vi "ReadSweepConfigurationFile.vi"(8 "error in (no error)":errorcluster, 10 "Path":path, 11 "SweepControl in":refnum<class "SweepControl.lvclass">) -> (0 "error out":errorcluster, 2 "Data":variant, 3 "SweepControl out":refnum<class "SweepControl.lvclass">)   [LabVIEW 2016, in "SweepControl.lvclass"]
uses:
  SweepControl.lvclass
  Transport/subVI/LockinVsg Configuration--Cluster.ctl
  Typedefs/Continuous B Sweep Configuration--Cluster.ctl
  Typedefs/Enum - Experiments.ctl
  Typedefs/Sweep Control Configuration--Cluster.ctl
  Typedefs/ScanControl.ctl
  Typedefs/Cluster - ScanControl.ctl
  Typedefs/Enum - Priority.ctl
  Typedefs/Enum - Action.ctl
  Typedefs/ScanParamters.ctl
  Typedefs/Cluster - ScanParamters.ctl
  <vilib>/addons/_JKI.lib/Serialization/JSON/JKI JSON Serialization.lvlib
  Transport/Transport.lvclass
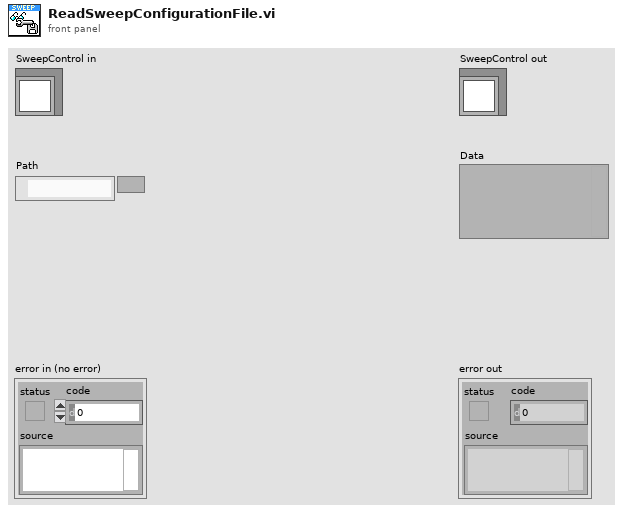
[diagram p1: front panel]
types:
  T1 = typedef "Transport.lvclass/LockinVsg Configuration--Cluster.ctl" = cluster{"Vsg Values":dbl[]}
  T2 = typedef "SweepControl.lvclass/Continuous B Sweep Configuration--Cluster.ctl" = cluster{"B field values":dbl[], "Experiment":T3}
  T3 = typedef "SweepControl.lvclass/Enum - Experiments.ctl" = enum16{"IV", "Lockin_time", "Lockin_Vsg", "Lockin (experimental)", "Lockin_Vsg_JKISM"}
  T4 = typedef "SweepControl.lvclass/Sweep Control Configuration--Cluster.ctl" = cluster{"Scan control":T5, "Scan parameters":T9, "Experiment":T3}
  T5 = typedef "SweepControl.lvclass/ScanControl.ctl" = T6[]
  T6 = typedef "SweepControl.lvclass/Cluster - ScanControl.ctl" = cluster{"Priority":T7, "Scan name":T8}
  T7 = typedef "SweepControl.lvclass/Enum - Priority.ctl" = enum16{"Priority 0", "Priority 1", "Priority 2", "Priority 3", "Priority 4", "Priority 5"}
  T8 = typedef "SweepControl.lvclass/Enum - Action.ctl" = enum16{"OFF", "DSA_Vamp", "DSA_freq", "DSA_Vsg1", "DSA_Vsg2", "DSA_Vsg3", "DAQ_Vbg", "B_Field", "Humidity", "Temp", "MW_freq1", "MW_freq2", "MW_amplitude1", "MW_amplitude2"}
  T9 = typedef "SweepControl.lvclass/ScanParamters.ctl" = T10[]
  T10 = typedef "SweepControl.lvclass/Cluster - ScanParamters.ctl" = cluster{"Start":dbl, "End":dbl, "Step":dbl, "Rate":dbl, "wait (ms)":u32, "Address":string, "channel":i32}
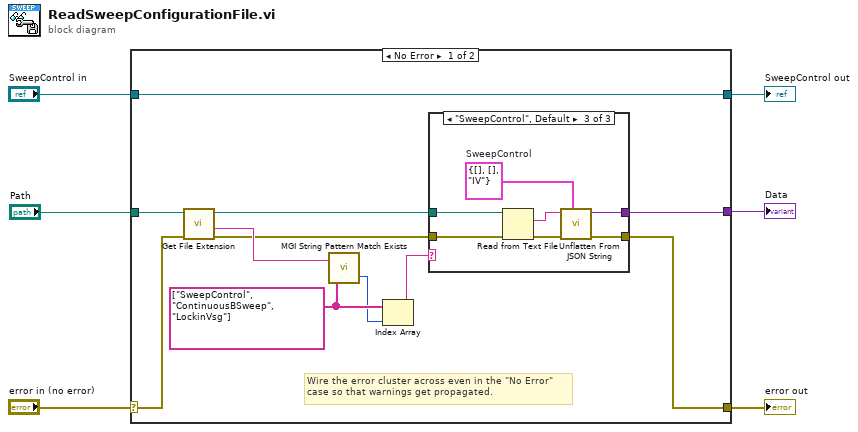
[diagram p0: block diagram]
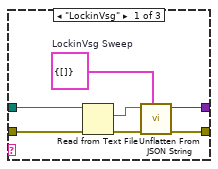
[diagram p2: hidden frame]
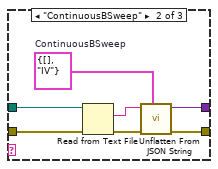
[diagram p3: hidden frame]
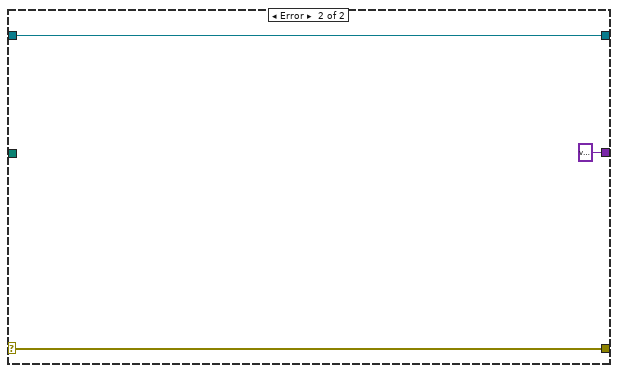
[diagram p4: hidden frame]
diagram:
  n1 = case shown="No Error" "error in (no error)" {
    selector: "error in (no error)" -> [w8 w41]
    tunnel: [w7 w41] -> w5
    tunnel: [w17 w40] -> w3
    tunnel: "SweepControl in" -> [w17 w40]
    tunnel: "Path" -> [w16 _]
    tunnel: [w9 variant ("Variant")] -> w1
    frame No Error {
      w14 = string[] ["SweepControl", "ContinuousBSweep", "LockinVsg"] ("Patterns to Try")
      # "Wire the error cluster across even in the \"No Error\"\ncase so that warnings get propagated."
      n2 = call <vilib>:"Get File Extension.vi"("error in (no error)"=w8, "file"=w16) -> ("error out"=w11:errorcluster, "filename without extension"=w13:string, "dup file"=w10:path)  [unwired: 5 in, 2 out]
      n3 = call <userlib>:"MGI String Pattern Match Exists.vi"("Patterns to Try"=w14, "String"=w13) -> ("Index of First Pattern Matched"=w12:i32)  [unwired: 1 out]
      n4 = Index Array(array=w14, index=w12) -> (element=w15:string)
      n5 = case shown="\"SweepControl\", Default" w15 {
        tunnel: w11 -> [w22 w29 w36]
        tunnel: w10 -> [w21 w28 w35]
        tunnel: [w19 w27 w34] -> w9
        tunnel: [w18 w26 w33] -> w7
        frame "LockinVsg" {
          w20 = T1 {"Vsg Values"=[]}  # LockinVsg Sweep
          n6 = Read from Text File(file (use dialog)=w21, error in=w22) -> (text=w23:string, error out=w24:errorcluster)  [unwired: 2 in, 2 out]
          n7 = call <vilib>:"Unflatten From JSON String.vi"("Type and Defaults"=w20, "error in (no error)"=w24, "JSON String"=w23) -> ("error out"=w18:errorcluster, "Variant"=w19:variant)  [unwired: 7 in]
        }
        frame "ContinuousBSweep" {
          w25 = T2 {"B field values"=[], "Experiment"=enum."IV"}  # ContinuousBSweep
          n8 = Read from Text File(file (use dialog)=w28, error in=w29) -> (text=w30:string, error out=w31:errorcluster)  [unwired: 2 in, 2 out]
          n9 = call <vilib>:"Unflatten From JSON String.vi"("Type and Defaults"=w25, "error in (no error)"=w31, "JSON String"=w30) -> ("error out"=w26:errorcluster, "Variant"=w27:variant)  [unwired: 7 in]
        }
        frame "SweepControl", Default {
          w32 = T4 {"Scan control"=[], "Scan parameters"=[], "Experiment"=enum."IV"}  # SweepControl
          n10 = Read from Text File(file (use dialog)=w35, error in=w36) -> (text=w37:string, error out=w38:errorcluster)  [unwired: 2 in, 2 out]
          n11 = call <vilib>:"Unflatten From JSON String.vi"("Type and Defaults"=w32, "error in (no error)"=w38, "JSON String"=w37) -> ("error out"=w33:errorcluster, "Variant"=w34:variant)  [unwired: 7 in]
        }
      }
    }
    frame Error {
    }
  }
  "error out" <- w5
  "SweepControl out" <- w3
  "Data" <- w1
